vi "arb_data.vi"(7 "name":string, 10 "wf":dbl[](array[numeric]), 11 "channel":u8=1) -> (2 "cmd":string)   [LabVIEW 2017, in "wf.lvlib"]
uses:
  wf.lvlib
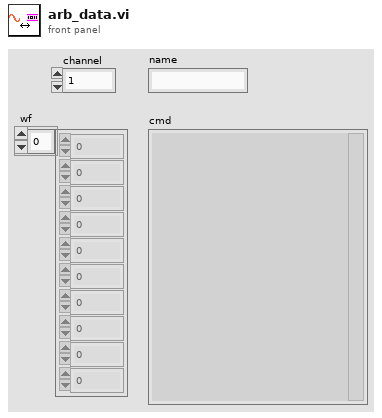
[diagram p1: front panel]
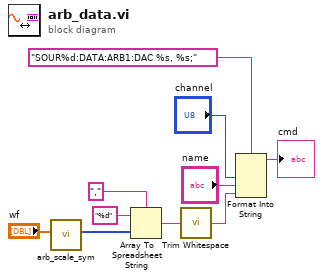
[diagram p0: block diagram]
diagram:
  n1 = call "arb_scale_sym.vi"("wf"="wf") -> ("data"=w6:i16[])  [unwired: 10 in]
  n2 = Array To Spreadsheet String(delimiter (Tab)=",", array=w6, 3:"%d" ("format string")) -> (spreadsheet string=w3:string)
  n3 = call <vilib>:"Trim Whitespace.vi"("string"=w3) -> ("trimmed string"=w2:string)  [unwired: 1 in]
  n4 = Format Into String(format string="SOUR%d:DATA:ARB1:DAC %s, %s;", "channel", "name", w2) -> (resulting string=→"cmd":string)  [unwired: 2 in, 1 out]
